vi "WSVCAP SHL Host LL SPI_RFFE Build Clock Rate and Wait Ticks.vi"(0 "Clock Rate (Hz)":dbl=50000.0, 7 "CMD Delay (s)":dbl[](array[numeric]) format="%#.3p s", 13 "Simulate FPGA":bool) -> (4 "Actual Rate (Hz)":dbl, 6 "Wait Ticks":u32, 8 "Actual Delay (s)":dbl[](array[numeric]) format="%#.0p s", 10 "CMD Delay (Ticks)":u32[](array[numeric]))   [LabVIEW 2017]
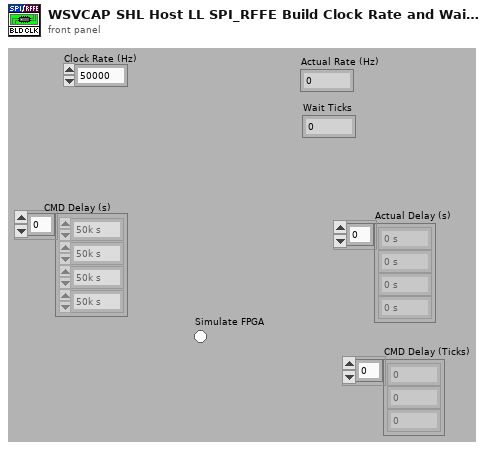
[diagram p1: front panel]
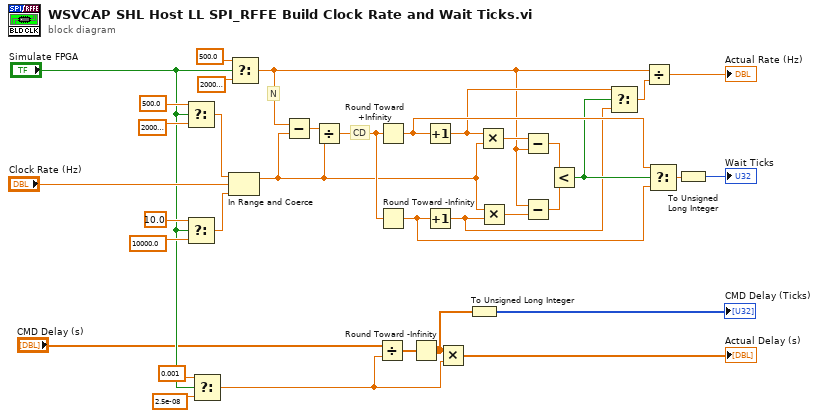
[diagram p0: block diagram]
diagram:
  # "CD"
  # "N"
  n1 = Select(t=500.0 ("10M"), s="Simulate FPGA", f=20000000.0 ("10M")) -> (s? t:f=w19:dbl)
  n2 = Select(t=10.0 ("10M"), s="Simulate FPGA", f=10000.0 ("10M")) -> (s? t:f=w18:dbl)
  n3 = Select(t=0.001 ("10M"), s="Simulate FPGA", f=2.5e-08 ("10M")) -> (s? t:f=w4:dbl)
  n4 = In Range and Coerce(upper limit=w19, x="Clock Rate (Hz)", lower limit=w18) -> (coerced(x)=w13:dbl)  [unwired: 1 out]
  n5 = Select(t=500.0 ("10M"), s="Simulate FPGA", f=20000000.0 ("10M")) -> (s? t:f=w21:dbl)
  n6 = Subtract(x=w21, y=w13) -> (x-y=w31:dbl)
  n7 = Divide(x=w31, y=w13) -> (x/y=w30:dbl)
  n8 = Divide(x="CMD Delay (s)", y=w4) -> (x/y=w5:dbl[])
  n9 = Round Toward +Infinity(x=w30) -> (ceil(x): smallest int >= x=w29:dbl)
  n10 = Round Toward -Infinity(1:w30) -> (0:w28:dbl)
  n11 = Round Toward -Infinity(1:w5) -> (0:w3:dbl[])
  n12 = Increment(x=w29) -> (x+1=w24:dbl)
  n13 = Increment(x=w28) -> (x+1=w25:dbl)
  n14 = Multiply(x=w3, y=w4) -> (x*y=→"Actual Delay (s)":dbl[])
  n15 = To Unsigned Long Integer(number=w3) -> (unsigned 32bit integer=→"CMD Delay (Ticks)":u32[])
  n16 = Multiply(x=w24, y=w13) -> (x*y=w35:dbl)
  n17 = Multiply(x=w13, y=w25) -> (x*y=w34:dbl)
  n18 = Subtract(x=w35, y=w21) -> (x-y=w32:dbl)
  n19 = Subtract(x=w21, y=w34) -> (x-y=w33:dbl)
  n20 = Less?(x=w32, y=w33) -> (x < y?=w26:bool)
  n21 = Select(t=w24, s=w26, f=w25) -> (s? t:f=w27:dbl)
  n22 = Divide(x=w21, y=w27) -> (x/y=→"Actual Rate (Hz)":dbl)
  n23 = Select(t=w29, s=w26, f=w28) -> (s? t:f=w20:dbl)
  n24 = To Unsigned Long Integer(number=w20) -> (unsigned 32bit integer=→"Wait Ticks":u32)
